vi "InsertOne.vi"(8 "error in (no error)":errorcluster, 10 "JSONString":string, 11 "MongoDB-Collection in":refnum<class "MongoDB-Collection.lvclass">) -> (0 "error out":errorcluster, 3 "MongoDB-Collection out":refnum<class "MongoDB-Collection.lvclass">)   [LabVIEW 2016, in "MongoDB-Collection.lvlib" / "MongoDB-Collection.lvclass"]
uses:
  MongoDB-Collection.lvclass
  D:/Users/blume/Desktop/LV/MongoDB-Driver/MLV DLLs/MongoLabVIEW.dll
  LV/MongoDB-Driver/MLV DLLs/MongoLabVIEW.dll
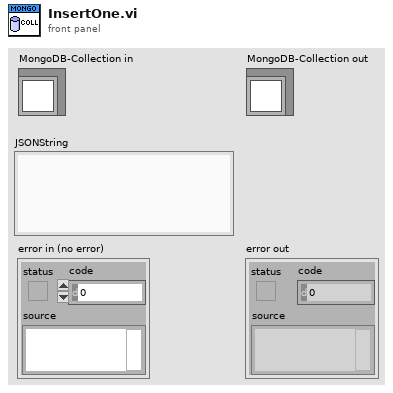
[diagram p1: front panel]
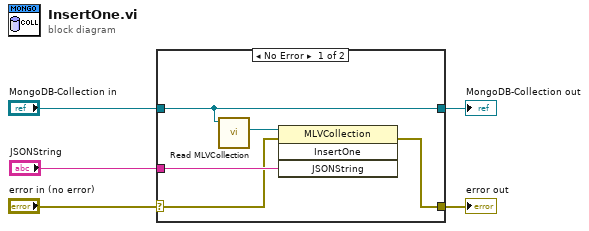
[diagram p0: block diagram]
diagram:
  n1 = case shown="No Error" "error in (no error)" {
    selector: "error in (no error)" -> [w7 w12]
    tunnel: [w6 w12] -> w4
    tunnel: [w10 w11] -> w2
    tunnel: "MongoDB-Collection in" -> [w10 w11]
    tunnel: "JSONString" -> [w8 _]
    frame No Error {
      n2 = call "Read MLVCollection.vi"("MongoDB-Collection in"=w10) -> ("MLVCollection"=w9:refnum<k24>)  [unwired: 8 in, 2 out]
      n3 = invoke class="MLVCollection" method="InsertOne"(reference=w9, error in=w7, "JSONString"=w8) -> (error out=w6:errorcluster)  [unwired: 1 in, 3 out]
    }
    frame Error {
    }
  }
  "error out" <- w4
  "MongoDB-Collection out" <- w2
